vi "manual test.vi"() -> ()   [LabVIEW 2013, in "alarms module tests.lvlib"]
uses:
  alarms module tests.lvlib
  module/configuration/alarms module configuration.lvclass
  module/execution/alarms module runtime.lvclass
  module/configuration/alarm configuration.ctl
  module/configuration/alarm comparison.ctl
  <vilib>/NI/Tag Bus Module Framework/channel/TBM channel.lvclass
  module/configuration/compare type.ctl
  module/configuration/boolean operation.ctl
  <vilib>/NI/Tag Bus/tag/Data Type.ctl
  <vilib>/NI/Tag Bus Module Framework/channel/channel classification.ctl
  module/configuration/alarms module configuration.lvclass/alarms module configuration.ctl
  <vilib>/NI/Tag Bus/tag/tag descriptor.lvclass/tag descriptor.ctl
  <vilib>/NI/Tag Bus/table/data polymorphs/write one/write Boolean.vi
  <vilib>/NI/Tag Bus/table/data polymorphs/write one/write Double.vi
  <vilib>/NI/Tag Bus/table/data polymorphs/write one/write U64.vi
  <vilib>/NI/Tag Bus/table/data polymorphs/read one/read Boolean.vi
  module/configuration/Write alarms.vi
  <vilib>/NI/Tag Bus/tag/read tag name.vi
  <vilib>/NI/Tag Bus/tag/read data type.vi
  <vilib>/NI/Tag Bus/dictionary/locate tag.vi
  <vilib>/NI/Configuration Framework/serializable configuration/NISE_CEF_serializable configuration.lvclass
  <vilib>/NI/Tag Bus/tag/tag descriptor.lvclass
  <vilib>/NI/Tag Bus/dictionary/data dictionary.lvclass
  <vilib>/NI/Tag Bus/table/data table.lvlib
panel:
  in  "enable latching":bool
  in  "a":dbl
  in  "b":u64
  in  "unlatch":bool
  in  "stop":bool
  out "out":bool
  out "final error":errorcluster
  out "output error":errorcluster
  out "input lookup error":errorcluster
  out "init error":errorcluster
  out "correct execution settings":bool
  out "serialization problem":errorcluster
  out "invalid configuration":errorcluster
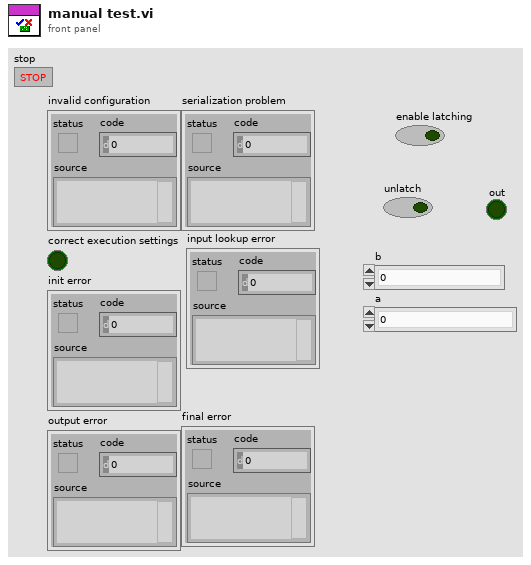
[diagram p1: front panel]
types:
  T1 = typedef "TBM channel.lvclass/channel classification.ctl" = enum16{"input data", "output data", "processing parameter", "processing result"}
  T2 = typedef "tag bus.lvlib/tag descriptor.lvclass/Data Type.ctl" = enum16{"Double", "Single", "I64", "I32", "I16", "I8", "U64", "U32", "U16", "U8", "Boolean", "String", "Array of Double", "Array of Single", "Array of I64", "Array of I32", "Array of I16", "Array of I8", "Array of U64", "Array of U32", "Array of U16", "Array of U8", "Array of Boolean", "Array of String"}
  T3 = typedef "alarms module configuration.lvclass/compare type.ctl" = enum16{">", "<", ">=", "<=", "="}
  T4 = typedef "alarms module configuration.lvclass/boolean operation.ctl" = enum16{"AND", "OR"}
  T5 = typedef "alarms module configuration.lvclass/alarm comparison.ctl" = cluster{"input channel":refnum<class "TBM channel.lvclass">, "limit":dbl, "comparison":T3}
  T6 = typedef "alarms module configuration.lvclass/alarm configuration.ctl" = cluster{"alarm name":string, "comparisons":T5[], "unlatch":refnum<class "TBM channel.lvclass">, "output":refnum<class "TBM channel.lvclass">, "boolean op":T4}
  T7 = typedef "TBM channel.lvclass/data tables.ctl" = cluster{"input data":T8, "processing parameter":T8, "processing result":T8, "output data":T8}
  T8 = typedef "tag bus.lvlib/dictionary table pair.ctl" = cluster{"data dictionary":refnum<class "data dictionary.lvclass">, "data table":T9}
  T9 = typedef "tag bus.lvlib/data table.lvlib/data table.ctl" = cluster{"Double":dbl[], "Single":sgl[], "I64":i64[], "I32":i32[], "I16":i16[], "I8":i8[], "U64":u64[], "U32":u32[], "U16":u16[], "U8":u8[], "Boolean":bool[], "String":string[], "Array of Double":cluster{"DBL Array":dbl[]}[], "Array of Single":cluster{"SGL Array":sgl[]}[], "Array of I64":cluster{"I64 Array":i64[]}[], "Array of I32":cluster{"I32 Array":i32[]}[], "Array of I16":cluster{"I16 Array":i16[]}[], "Array of I8":cluster{"I8 Array":i8[]}[], "Array of U64":cluster{"U64 Array":u64[]}[], "Array of U32":cluster{"U32 Array":u32[]}[], "Array of U16":cluster{"U16 Array":u16[]}[], "Array of U8":cluster{"U8 Array":u8[]}[], "Array of Boolean":cluster{"Boolean Array":bool[]}[], "Array of String":cluster{"String Array":string[]}[]}
  T10 = typedef "TBM module execution interface.lvclass/execution settings.ctl" = cluster{"reads inputs":bool, "processes data":bool, "writes outputs":bool}
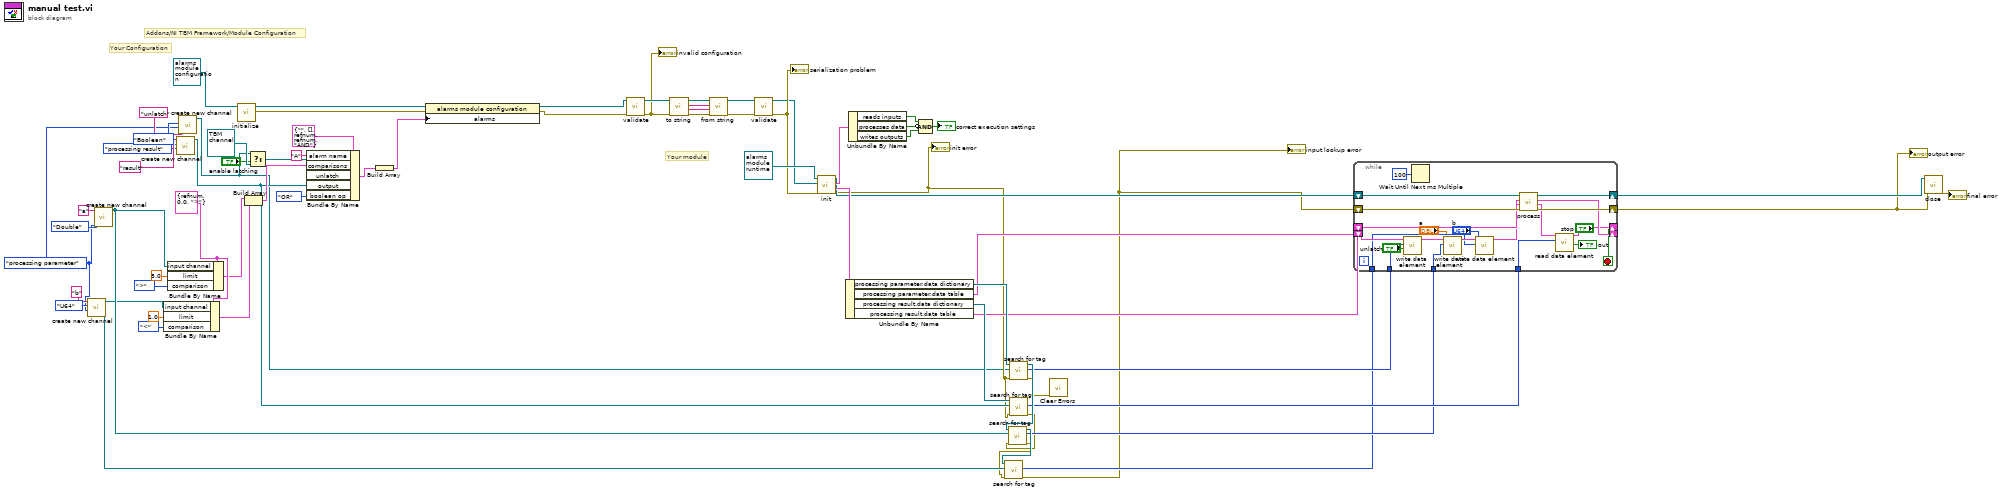
[diagram p0: block diagram]
diagram:
  w26 = channel_classification."processing parameter" ("channel classification")
  w36 = Data_Type."Boolean" ("data type")
  w44 = T5 {"input channel"=refnum, "limit"=0.0, "comparison"=enum.">"} ("alarm cfg")
  # "Your module"
  # "Your Configuration"
  # "Addons/NI TBM Framework/Module Configuration"
  n1 = call <vilib>:"create new channel.vi"("channel classification"=w26, "data type"=Data_Type."U64", "channel name"="b") -> ("channel"=w20:refnum<class "TBM channel.lvclass">)  [unwired: 8 in]
  n2 = call <vilib>:"create new channel.vi"("channel classification"=w26, "data type"=Data_Type."Double", "channel name"="a") -> ("channel"=w21:refnum<class "TBM channel.lvclass">)  [unwired: 8 in]
  n3 = Bundle By Name(cluster=w44, "input channel"=w20, "limit"=1.0, "comparison"=compare_type."<") -> (w42:T5)
  n4 = Bundle By Name(cluster=w44, "input channel"=w21, "limit"=5.0, "comparison"=compare_type.">") -> (w43:T5)
  n5 = call <vilib>:"create new channel.vi"("channel classification"=channel_classification."processing result", "data type"=w36, "channel name"="result") -> ("channel"=w22:refnum<class "TBM channel.lvclass">)  [unwired: 8 in]
  n6 = call <vilib>:"create new channel.vi"("channel classification"=w26, "data type"=w36, "channel name"="unlatch") -> ("channel"=w3:refnum<class "TBM channel.lvclass">)  [unwired: 8 in]
  n7 = call <vilib>:"initialize.vi"("configuration in"=refnum<class "alarms module configuration.lvclass"> refnum ("tag bus configurable plugin module configuration")) -> ("error out"=w51:errorcluster, "configuration out"=w50:refnum<class "alarms module configuration.lvclass">)  [unwired: 8 in, 1 out]
  n8 = Build Array(w43, w42) -> (w41:T5[])
  n9 = Select(t=w3, s="enable latching", f=refnum<class "TBM channel.lvclass"> refnum ("unlatch")) -> (s? t:f=w2:refnum<class "TBM channel.lvclass">)
  n10 = Bundle By Name(cluster=T6 {"alarm name"="", "comparisons"=[], "unlatch"=refnum, "output"=refnum, "boolean op"=enum."AND"} ("alarm config"), "alarm name"="A" ("comparison"), "comparisons"=w41, "unlatch"=w2, "output"=w22, "boolean op"=boolean_operation."OR") -> (w46:T6)
  n11 = Build Array(w46) -> (w45:T6[])
  n12 = property class="alarms module configuration"(reference=w50, error in=w51, "alarms"=w45) -> (reference out=w48:refnum<class "alarms module configuration.lvclass">, error out=w49:errorcluster)
  n13 = call-dynamic "validate.vi"("error in"=w49, "alarms module configuration in"=w48) -> ("error out"=w69:errorcluster, "alarms module configuration out"=w70:refnum<class "alarms module configuration.lvclass">)  [unwired: 8 in]
  "invalid configuration" <- w69
  n14 = call-dynamic "to string.vi"("error in"=w69, "alarms module configuration in"=w70) -> ("error out"=w65:errorcluster, "data"=w66:string, "version"=w67:string, "alarms module configuration out"=w68:refnum<class "alarms module configuration.lvclass">)  [unwired: 6 in]
  n15 = call-dynamic "from string.vi"("error in"=w65, "data"=w66, "version"=w67, "alarms module configuration in"=w68) -> ("error out"=w63:errorcluster, "alarms module configuration out"=w64:refnum<class "alarms module configuration.lvclass">)  [unwired: 6 in]
  n16 = call-dynamic "validate.vi"("error in"=w63, "alarms module configuration in"=w64) -> ("error out"=w61:errorcluster, "alarms module configuration out"=w60:refnum<class "alarms module configuration.lvclass">)  [unwired: 8 in]
  "serialization problem" <- w61
  n17 = call-dynamic "init.vi"("error in"=w61, "TBM module configuration in"=w60, "alarms module runtime in"=refnum<class "alarms module runtime.lvclass"> refnum ("tag bus configurable plugin module")) -> ("error out"=w6:errorcluster, "data allocations"=w54:T7, "execution settings"=w59:T10, "alarms module runtime out"=w25:refnum<class "alarms module runtime.lvclass">)  [unwired: 5 in]
  "init error" <- w6
  n18 = Unbundle By Name(w54) -> ("processing parameter.data dictionary"=w19:refnum<class "data dictionary.lvclass">, "processing parameter.data table"=w15:T9, "processing result.data dictionary"=w16:refnum<class "data dictionary.lvclass">, "processing result.data table"=w14:T9)
  n19 = Unbundle By Name(w59) -> ("reads inputs"=w56:bool, "processes data"=w58:bool, "writes outputs"=w57:bool)
  n20 = Compound Arithmetic op=AND(w56, invert w58, w57) -> (→"correct execution settings":bool)
  n21 = call <vilib>:"search for tag.vi"("error in"=w6, "system tag"=w3, "data dictionary in"=w19) -> ("error out"=w5:errorcluster, "index"=w12:i32, "data dictionary out"=w18:refnum<class "data dictionary.lvclass">)  [unwired: 6 in]
  n22 = call <vilib>:"search for tag.vi"("error in"=w6, "system tag"=w22, "data dictionary in"=w16) -> ("error out"=w9:errorcluster, "index"=w13:i32)  [unwired: 6 in, 1 out]
  n23 = call <vilib>:"search for tag.vi"("error in"=w9, "system tag"=w21, "data dictionary in"=w18) -> ("error out"=w8:errorcluster, "index"=w11:i32, "data dictionary out"=w17:refnum<class "data dictionary.lvclass">)  [unwired: 6 in]
  n24 = call <vilib>:"search for tag.vi"("error in"=w8, "system tag"=w20, "data dictionary in"=w17) -> ("error out"=w7:errorcluster, "index"=w10:i32)  [unwired: 6 in, 1 out]
  "input lookup error" <- w7
  n25 = call <vilib>:"Clear Errors.vi"("error in (no error)"=w5) -> ()  [unwired: 6 in, 1 out]
  n26 = while {
    shift-right: [w91] -> w24
    shift-left: w25 -> [w92]
    shift-right: [w89] -> w23
    shift-left: w7 -> [w90]
    shift-right: [w88] -> _
    shift-left: w15 -> [w84]
    shift-right: [w81] -> _
    shift-left: w14 -> [w87]
    tunnel: w13 -> [w80]
    tunnel: w12 -> [w76]
    tunnel: w11 -> [w74]
    tunnel: w10 -> [w73]
    stop <- "stop" stop-if-true
    n27 = call-poly <vilib>:"write data element.vi"("value"="unlatch", "index"=w76, "data table in"=w84) -> ("data table out"=w85:T9)  [unwired: 8 in]
    n28 = Wait Until Next ms Multiple(millisecond multiple=u32 100) -> ()  [unwired: 1 out]
    n29 = call-poly <vilib>:"write data element.vi"("value"="a", "index"=w74, "data table in"=w85) -> ("data table out"=w86:T9)  [unwired: 8 in]
    n30 = call-poly <vilib>:"write data element.vi"("value"="b", "index"=w73, "data table in"=w86) -> ("data table out"=w83:T9)  [unwired: 8 in]
    n31 = call-dynamic "process.vi"("error in"=w90, "result allocation"=w87, "parameters"=w83, "module in"=w92) -> ("error out"=w89:errorcluster, "results"=w82:T9, "parameter allocation"=w88:T9, "module out"=w91:refnum<class "alarms module runtime.lvclass">)  [unwired: 4 in]
    n32 = call-poly <vilib>:"read data element.vi"("index"=w80, "data table in"=w82) -> ("value"=→"out":bool, "data table out"=w81:T9)  [unwired: 8 in]
  }
  "output error" <- w23
  n33 = call-dynamic "close.vi"("error in"=w23, "alarms module runtime in"=w24) -> ("error out"=→"final error":errorcluster)  [unwired: 9 in]
